vi "FormatFailureMessage.vi"(8 "error in (no error)":errorcluster, 10 "Restricted Object":string, 11 "VI Name":string) -> (0 "error out":errorcluster, 2 "Output/Failure":string)   [LabVIEW 2014, in "BuildSecurity.lvlib"]
doc: "Sets the output message based on the provided blacklisted object."
uses:
  BuildSecurity.lvlib
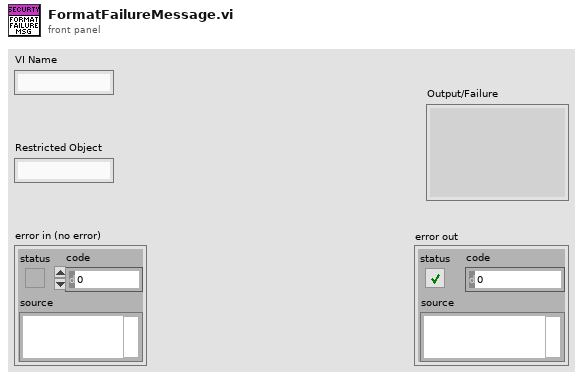
[diagram p1: front panel]
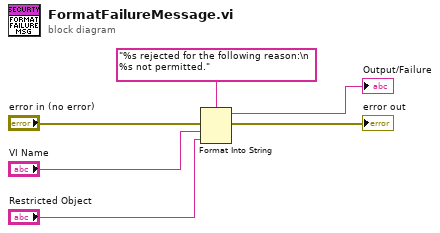
[diagram p0: block diagram]
diagram:
  n1 = Format Into String(format string="%s rejected for the following reason:\n   %s not permitted.", error in="error in (no error)", "VI Name", "Restricted Object") -> (resulting string=→"Output/Failure":string, error out=→"error out":errorcluster)  [unwired: 1 in]
